vi "Comments.Create Lockin REF Description.vi"(7 "error in (no error)":errorcluster, 10 "Control Experiment":refnum<class "Control Experiment SM.lvclass">) -> (0 "error out":errorcluster, 2 "REF Section":string, 3 "Control Experiment out":refnum<class "Control Experiment SM.lvclass">)   [LabVIEW 2016, in "Control Experiment SM.lvclass"]
uses:
  Control Experiment SM.lvclass
  <userlib>/LevyLab/Lockin-Multichannel/Instrument.Lockin/Instrument.Lockin.lvclass
  <userlib>/LevyLab/PLYM/YAML.lvclass
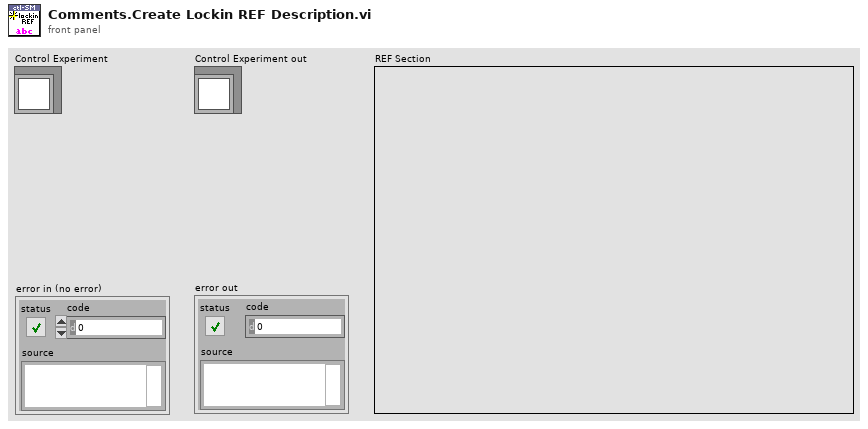
[diagram p1: front panel]
types:
  T1 = typedef "Lockin.DAQ.lvclass/REF-cluster.ctl" = cluster{"Ch":i32[], " f (Hz)":dbl[], "Phase (°)":dbl[], "TC (s)":dbl[], "order":i32[]}
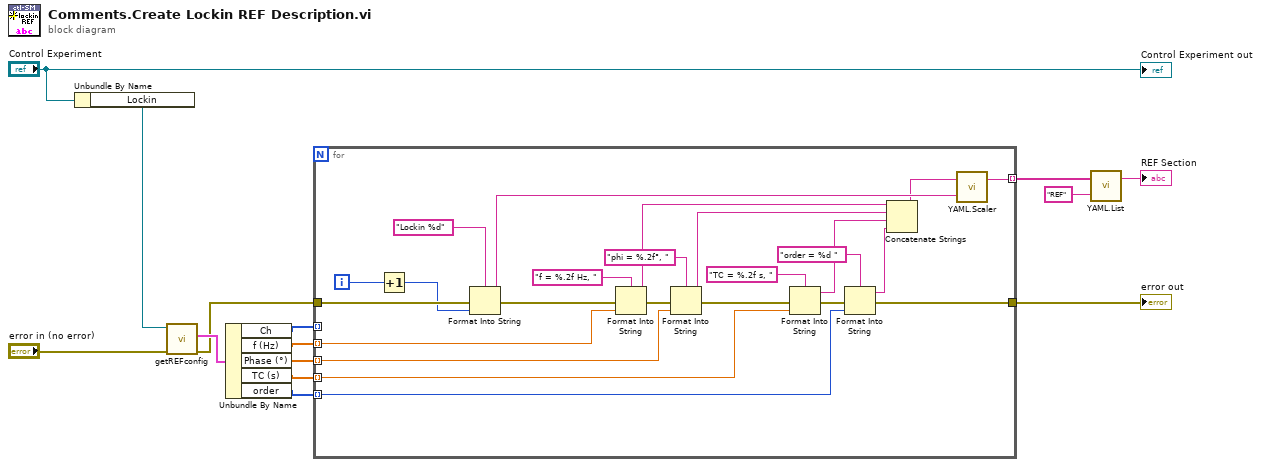
[diagram p0: block diagram]
diagram:
  n1 = Unbundle By Name("Control Experiment") -> ("Lockin"=w5:refnum<class "Instrument.Lockin.lvclass">)
  n2 = call <userlib>:"getREFconfig.vi"("error in (no error)"="error in (no error)", "Instrument.Lockin in"=w5) -> ("error out"=w4:errorcluster, "REFconfig"=w6:T1)  [unwired: 7 in, 1 out]
  n3 = Unbundle By Name(w6) -> ("Ch"=w14:i32[], "f (Hz)"=w13:dbl[], "Phase (°)"=w3:dbl[], "TC (s)"=w2:dbl[], "order"=w1:i32[])
  n4 = for {
    tunnel: w14 -> [_] mode=indexing
    tunnel: w13 -> [w24] mode=indexing
    tunnel: w4 -> [w38]
    tunnel: [w19] -> w12
    tunnel: [w27] -> w7 mode=indexing
    tunnel: w3 -> [w25] mode=indexing
    tunnel: w2 -> [w18] mode=indexing
    tunnel: w1 -> [w17] mode=indexing
    i -> [w36]
    n5 = Increment(x=w36) -> (x+1=w26:i32)
    n6 = Format Into String(format string="Lockin %d", error in=w38, w26) -> (resulting string=w29:string, error out=w31:errorcluster)  [unwired: 1 in]
    n7 = Format Into String(format string="f = %.2f Hz, ", error in=w31, w24) -> (resulting string=w33:string, error out=w37:errorcluster)  [unwired: 1 in]
    n8 = Format Into String(format string="phi = %.2f°, ", error in=w37, w25) -> (resulting string=w32:string, error out=w20:errorcluster)  [unwired: 1 in]
    n9 = Format Into String(format string="TC = %.2f s, ", error in=w20, w18) -> (resulting string=w15:string, error out=w21:errorcluster)  [unwired: 1 in]
    n10 = Format Into String(format string="order = %d ", error in=w21, w17) -> (resulting string=w16:string, error out=w19:errorcluster)  [unwired: 1 in]
    n11 = Concatenate Strings(w33, w32, w15, w16) -> (w28:string)
    n12 = call <userlib>:"YAML.Scaler.vi"("Key"=w29, "Scaler"=w28) -> ("Output"=w27:string)  [unwired: 1 in]
  }
  "error out" <- w12
  n13 = call <userlib>:"YAML.List.vi"("Key"="REF" ("string"), "lines"=w7) -> ("Output"=→"REF Section":string)  [unwired: 1 in]
  "Control Experiment out" <- "Control Experiment"
